vi "Renishaw-XL80_SetExpansionCoefficient.vi"(8 "error in (no error)":errorcluster, 10 "ExpansionCoefficient":dbl, 11 "Renishaw-XL80 in":refnum<class "Renishaw-XL80.lvclass">) -> (0 "error out":errorcluster, 3 "Renishaw-XL80 out":refnum<class "Renishaw-XL80.lvclass">)   [LabVIEW 2024, in "Renishaw-XL80.lvclass"]
doc: "Writing this property will set the material expansion coefficient in ppm/°C.\n\nDefinition\nHRESULTput_ExpansionCoefficient( [in] double newVal);\nParameters\nnewVal\nSpecifies the material expansion coefficient to use in ppm/°C.\n\nComments\nWriting this property always succeeds. It will return an HRESULT of S_OK.\n\nIf the client has set AutoCompensationMode to AUTO_COMPENSATION_FULL then setting this property will also update the material compensation factor."
uses:
  Renishaw-XL80.lvclass
  Renishaw-XL80.lvclass/Renishaw-XL80.ctl
  D:/A.C.M/Example CSharp_64/bin/Debug/Interop.DX10SDKADAPTORLib.dll
  Example CSharp_64/bin/Debug/Interop.DX10SDKADAPTORLib.dll
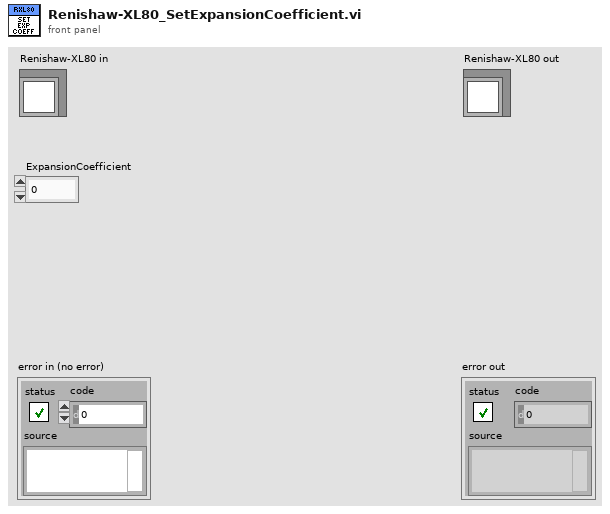
[diagram p1: front panel]
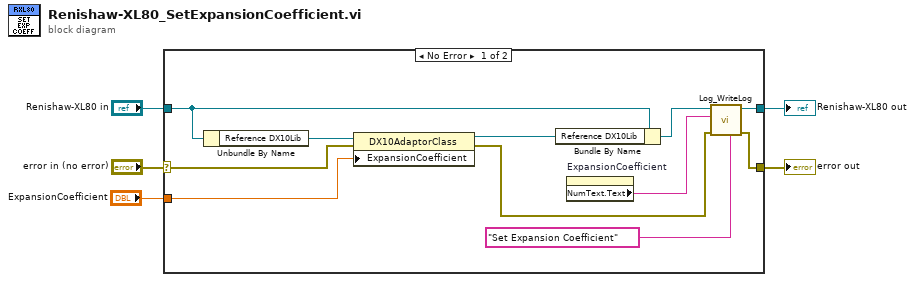
[diagram p0: block diagram]
diagram:
  n1 = case shown="No Error" "error in (no error)" {
    selector: "error in (no error)" -> [w13 w18]
    tunnel: [w8 w18] -> w4
    tunnel: [w10 w17] -> w2
    tunnel: "Renishaw-XL80 in" -> [w14 w17]
    tunnel: "ExpansionCoefficient" -> [w12 _]
    frame No Error {
      n2 = Unbundle By Name(w14) -> ("Reference DX10Lib"=w16:refnum<k24>)
      n3 = property class="DX10AdaptorClass"(reference=w16, error in=w13, "ExpansionCoefficient"=w12) -> (reference out=w15:refnum<k24>, error out=w6:errorcluster)
      n4 = Bundle By Name(cluster=w14, "Reference DX10Lib"=w15) -> (w11:refnum<class "Renishaw-XL80.lvclass">)
      n5 = property on="ExpansionCoefficient" class="DigNum (strict)"() -> ("NumText.Text"=w9:string)  [unwired: 2 in, 2 out]
      n6 = call-dynamic "Log_WriteLog.vi"("Additional text"="Set Expansion Coefficient", "error in (no error)"=w6, "Command"=w9, "Log in"=w11) -> ("error out"=w8:errorcluster, "Log out"=w10:refnum<class "Renishaw-XL80.lvclass">)  [unwired: 6 in]
    }
    frame Error {
    }
  }
  "error out" <- w4
  "Renishaw-XL80 out" <- w2
